vi "tm486_dataextraction_toDCIMG.vi"() -> ()   [LabVIEW 2021]
panel:
  in  "r1 oy":i32
  in  "r1 sx":i32=512
  in  "r1 sy":i32=512
  in  "r1 ox":i32
  in  "r2 oy":i32=1024
  in  "r2 ox":i32=1024
  in  "r2 sx":i32=512
  in  "r2 sy":i32=512
  out "Frames Recorded":i32
  in  "DCIMG Path":path
  in  "Frames":i32=100
  out "Error Out":errorcluster
  # "This is an example of how to use the\nhard disk recorder functions to record\nimages to a DCIMG file."
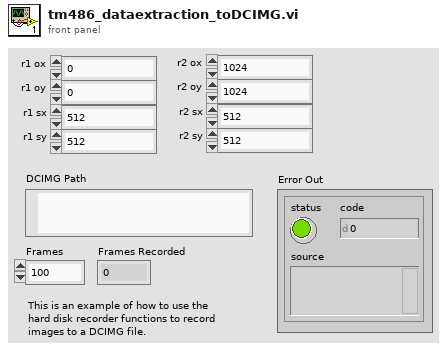
[diagram p1: front panel]
types:
  T1 = cluster{"r1 ox":i32, "r1 oy":i32, "r1 sx":i32, "r1 sy":i32}
  T2 = cluster{"r2 ox":i32, "r2 oy":i32, "r2 sy":i32, "r2 sx":i32}
  T3 = cluster{"r2 ox":i32, "r2 oy":i32, "r2 sy":i32, "r2 sx":i32}[]
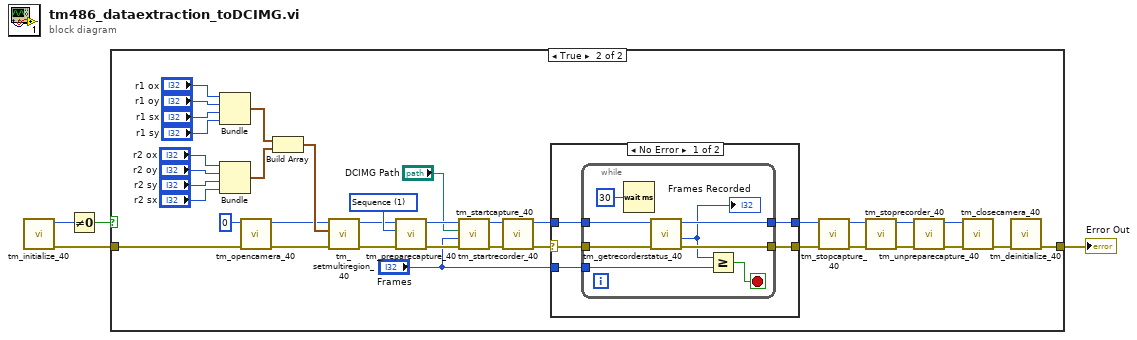
[diagram p0: block diagram]
diagram:
  n1 = call <userlib>:"tm_initialize_40.vi"() -> ("error out"=w1:errorcluster, "Number Of Cameras"=w2:u32)  [unwired: 8 in, 2 out]
  n2 = Not Equal To 0?(x=w2) -> (x != 0?=w4:bool)
  n3 = case shown="True" w4 {
    tunnel: w1 -> [w5 w41]
    tunnel: [w5 w37] -> w3
    frame False {
    }
    frame True {
      w39 = 1 items=["Snap", "Sequence"] ("Capture mode")
      n4 = Bundle("r1 ox"="r1 ox", "r1 oy"="r1 oy", "r1 sx"="r1 sx", "r1 sy"="r1 sy") -> (w18:T1)  [unwired: 1 in]
      n5 = Bundle("r2 ox"="r2 ox", "r2 oy"="r2 oy", "r2 sy"="r2 sy", "r2 sx"="r2 sx") -> (w10:T2)  [unwired: 1 in]
      n6 = call <userlib>:"tm_opencamera_40.vi"("error in (no error)"=w41, "Camera Index"=u32 0) -> ("error out"=w6:errorcluster, "Handle out"=w7:u32)  [unwired: 7 in, 1 out]
      n7 = Build Array(w18, w10) -> (w15:T3)
      n8 = call <userlib>:"tm_setmultiregion_40.vi"("error in (no error)"=w6, "Sub Regions"=w15, "Handle in"=w7) -> ("error out"=w8:errorcluster, "Handle out"=w9:u32)  [unwired: 7 in]
      n9 = call <userlib>:"tm_preparecapture_40.vi"("error in (no error)"=w8, "Capture mode"=w39, "Handle in"=w9) -> ("error out"=w34:errorcluster, "Handle out"=w33:u32)  [unwired: 5 in, 2 out]
      n10 = call <userlib>:"tm_startrecorder_40.vi"("error in (no error)"=w34, "frames"="Frames", "File"="DCIMG Path", "Handle in"=w33) -> ("error out"=w32:errorcluster, "Handle out"=w31:u32)  [unwired: 6 in]
      n11 = call <userlib>:"tm_startcapture_40.vi"("error in (no error)"=w32, "Handle in"=w31) -> ("error out"=w30:errorcluster, "Handle out"=w29:u32)  [unwired: 8 in]
      n12 = case shown="No Error" w30 {
        selector: w30 -> [w46 w55]
        tunnel: w29 -> [w45 w56]
        tunnel: [w43 w56] -> w24
        tunnel: [w42 w55] -> w23
        tunnel: "Frames" -> [w44 _]
        frame No Error {
          n13 = while {
            tunnel: w46 -> [w52]
            tunnel: w45 -> [w51]
            tunnel: [w50] -> w42
            tunnel: [w53] -> w43
            tunnel: w44 -> [w54]
            stop <- w47 stop-if-true
            n14 = Wait (ms)(milliseconds to wait=u32 30) -> ()  [unwired: 1 out]
            n15 = call <userlib>:"tm_getrecorderstatus_40.vi"("error in (no error)"=w52, "Handle"=w51) -> ("error out"=w50:errorcluster, "Count"=w49:i32, "Handle"=w53:u32)  [unwired: 6 in, 1 out]
            "Frames Recorded" <- w49
            n16 = Greater Or Equal?(x=w49, y=w54) -> (x >= y?=w47:bool)
          }
        }
        frame Error {
        }
      }
      n17 = call <userlib>:"tm_stopcapture_40.vi"("error in (no error)"=w23, "Handle in"=w24) -> ("error out"=w21:errorcluster, "Handle out"=w22:u32)  [unwired: 8 in]
      n18 = call <userlib>:"tm_stoprecorder_40.vi"("error in (no error)"=w21, "Handle in"=w22) -> ("error out"=w25:errorcluster, "Handle out"=w26:u32)  [unwired: 8 in]
      n19 = call <userlib>:"tm_unpreparecapture_40.vi"("error in (no error)"=w25, "Handle in"=w26) -> ("error out"=w36:errorcluster, "Handle out"=w35:u32)  [unwired: 8 in]
      n20 = call <userlib>:"tm_closecamera_40.vi"("error in (no error)"=w36, "Handle in"=w35) -> ("error out"=w38:errorcluster)  [unwired: 9 in]
      n21 = call <userlib>:"tm_deinitialize_40.vi"("error in (no error)"=w38) -> ("error out"=w37:errorcluster)  [unwired: 10 in]
    }
  }
  "Error Out" <- w3
